vi "Mcp2210 Close.vi"(8 "error in (no error)":errorcluster, 11 "handle":i32) -> (0 "error out":errorcluster, 3 "handle out":i32)   [LabVIEW 2015, in "mcp2210.lvlib"]
doc: "Attempt to close a connection to a MCP2210.\nParameters:\nInputs:\n- IntPtr handle - Device handle we'll close the connection to.\nCannot be NULL nor contain invalid handle value.\nOutputs:\n- none\nReturns:\n- 0 for success: M_E_SUCCESS\n- negative error code: M_E_ERR_NULL, M_E_ERR_INVALID_HANDLE_VALUE\nM_E_ERR_CLOSE_FAILED\n\nMCP2210_DLL_UM_API int __stdcall Mcp2210_Close(void *handle);"
uses:
  <userlib>/mcp2210/mcp2210.lvlib
  <userlib>/mcp2210/mcp2210_dll_um_x86.dll
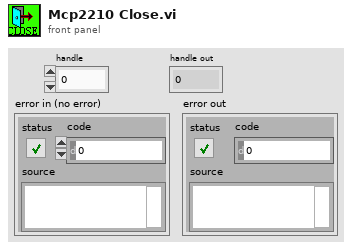
[diagram p1: front panel]
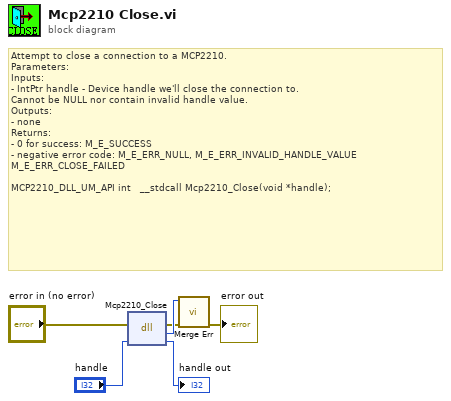
[diagram p0: block diagram]
diagram:
  # "Attempt to close a connection to a MCP2210.\nParameters:\nInputs:\n- IntPtr handle - Device handle we'll close the connection to.\nCannot be NULL nor contain invalid handle value.\nOutputs:\n- none\nReturns:\n- 0 for success: M_E_SUCCESS\n- negative error code: M_E_ERR_NULL, M_E_ERR_INVALID_HANDLE_VALUE\nM_E_ERR_CLOSE_FAILED\n\nMCP2210_DLL_UM_API int   __stdcall Mcp2210_Close(void *handle);"
  n1 = dll-call lib="D:/LabVIEW 2015/user.lib/mcp2210/mcp2210_dll_um_x86.*" fn="Mcp2210_Close"(error in="error in (no error)", "handle"="handle") -> (error out=w3:errorcluster, "return type"=w4:i32, "handle"=→"handle out":i32)  [unwired: 2 in, 1 out]
  n2 = call <userlib>:"Merge Err.vi"("error in (no error)"=w3, "return type"=w4) -> ("error out"=→"error out":errorcluster)  [unwired: 9 in]
